vi "Varint Array Decoder unit32 packed.vi"(7 "Optional":bool, 8 "error in":errorcluster, 9 "array in":u8[](array[numeric]), 10 "Key":i32=4) -> (0 "error out":errorcluster, 1 "array w/ subset deleted":u8[](array[numeric]), 3 "varint_array":u32[](array[numeric]))   [LabVIEW 2021]
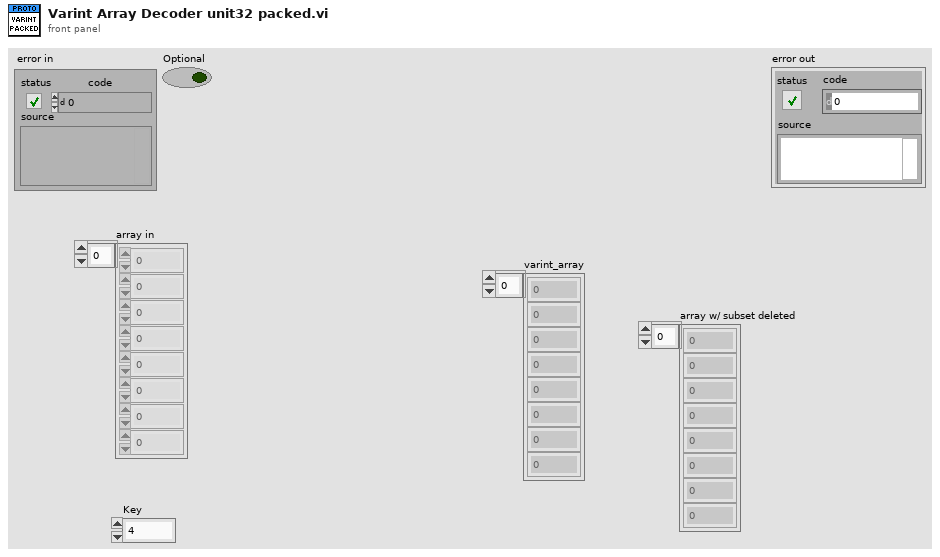
[diagram p1: front panel]
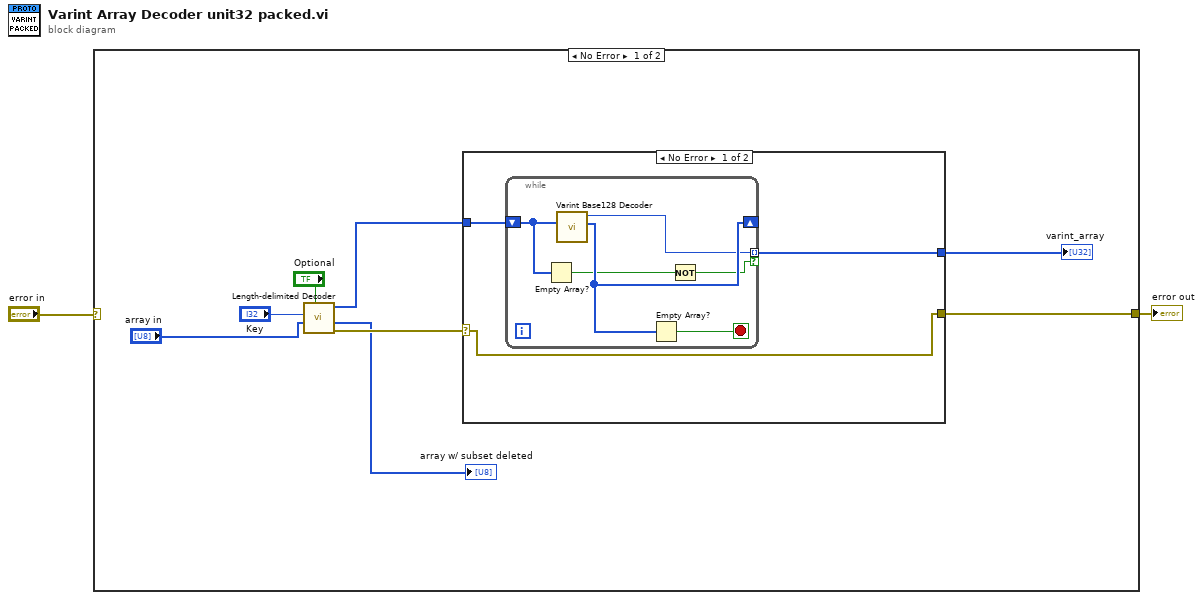
[diagram p0: block diagram]
diagram:
  n1 = case shown="No Error" "error in" {
    selector: "error in" -> [_ w21]
    tunnel: [w4 w21] -> w1
    frame No Error {
      n2 = call "Length-delimited Decoder.vi"("Optional"="Optional", "Array"="array in", "Key"="Key") -> ("error out"=w9:errorcluster, "array w/ subset deleted"=→"array w/ subset deleted":u8[], "Length-delimited"=w10:u8[])  [unwired: 5 in, 1 out]
      n3 = case shown="No Error" w9 {
        selector: w9 -> [w11 w20]
        tunnel: w10 -> [w13 _]
        tunnel: [w12 _] -> w8
        tunnel: [w11 w20] -> w4
        frame No Error {
          n4 = while {
            tunnel: [w17] -> w12 mode=indexing if=w14
            shift-right: [w18] -> _
            shift-left: w13 -> [w16]
            stop <- w19 stop-if-true
            n5 = Empty Array?(array=w16) -> (empty?=w15:bool)
            n6 = call "Varint Base128 Decoder.vi"("Array"=w16) -> ("array w/ subset deleted"=w18:u8[], "Numeric"=w17:i32)  [unwired: 9 in]
            n7 = Empty Array?(array=w18) -> (empty?=w19:bool)
            n8 = Not(x=w15) -> (.not. x?=w14:bool)
          }
        }
        frame Error {
        }
      }
      "varint_array" <- w8
    }
    frame Error {
    }
  }
  "error out" <- w1
